vi "Devices Processing.vi"(8 "error in (no error)":errorcluster, 10 "Devices":refnum<class "Device.lvclass">[](array[class]), 11 "SLMP in":refnum<class "SLMP.lvclass">) -> (0 "error out":errorcluster, 3 "SLMP out":refnum<class "SLMP.lvclass">)   [LabVIEW 2019, in "SLMP.lvlib" / "SLMP.lvclass"]
uses:
  SLMP.lvclass
  Device/Device.lvclass
  SLMP.lvclass/SLMP.ctl
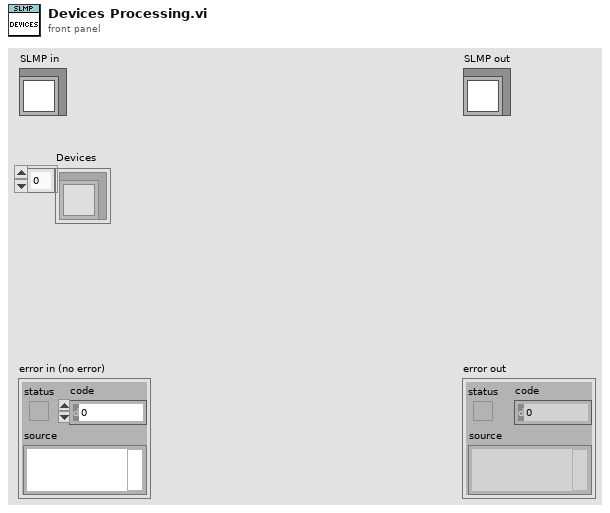
[diagram p1: front panel]
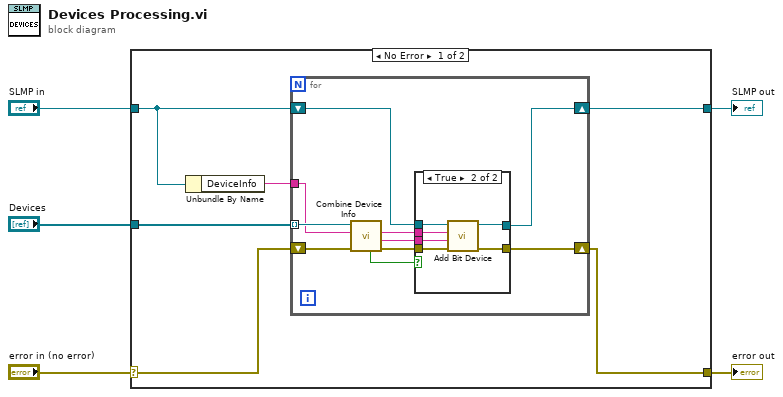
[diagram p0: block diagram]
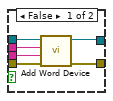
[diagram p2: hidden frame]
diagram:
  n1 = case shown="No Error" "error in (no error)" {
    selector: "error in (no error)" -> [w7 w35]
    tunnel: [w6 w35] -> w4
    tunnel: [w8 w34] -> w2
    tunnel: "SLMP in" -> [w9 w34]
    tunnel: "Devices" -> [w11 _]
    frame No Error {
      n2 = Unbundle By Name(w9) -> ("DeviceInfo"=w10:string)
      n3 = for {
        tunnel: w11 -> [w21] mode=indexing
        tunnel: w10 -> [w20]
        shift-right: [w15] -> w8
        shift-left: w9 -> [w16]
        shift-right: [w12] -> w6
        shift-left: w7 -> [w14]
        n4 = call "Combine Device Info.vi"("error in (no error)"=w14, "DeviceInfo"=w20, "Device in"=w21) -> ("error out"=w13:errorcluster, "Combined Device"=w17:string, "Device Code"=w18:string, "Bit Device?"=w19:bool)  [unwired: 4 in, 1 out]
        n5 = case shown="True" w19 {
          tunnel: w18 -> [w27 w33]
          tunnel: w17 -> [w24 w32]
          tunnel: w16 -> [w26 w31]
          tunnel: [w25 w30] -> w15
          tunnel: w13 -> [w23 w29]
          tunnel: [w22 w28] -> w12
          frame False {
            n6 = call "Add Word Device.vi"("error in (no error)"=w23, "Device <JSON>"=w24, "Device Code"=w27, "SLMP in"=w26) -> ("error out"=w22:errorcluster, "SLMP out"=w25:refnum<class "SLMP.lvclass">)  [unwired: 6 in]
          }
          frame True {
            n7 = call "Add Bit Device.vi"("error in (no error)"=w29, "Device <JSON>"=w32, "Device Code"=w33, "SLMP in"=w31) -> ("error out"=w28:errorcluster, "SLMP out"=w30:refnum<class "SLMP.lvclass">)  [unwired: 6 in]
          }
        }
      }
    }
    frame Error {
    }
  }
  "error out" <- w4
  "SLMP out" <- w2
